vi "DO Monitoring Global Variables.vi"() -> ()   [LabVIEW 2014]
panel:
  in  "OutPuts":T1(tab)
  out "View Out":T2
  out "View Out 2":T2
  out "View Out 3":T2
  out "View Out 4":T2
  out "View Out 5":T2
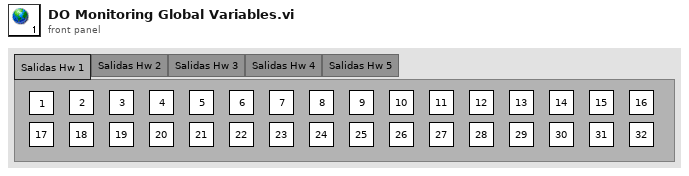
[diagram p1: front panel]
types:
  T1 = enum32{"Salidas Hw 1", "Salidas Hw 2", "Salidas Hw 3", "Salidas Hw 4", "Salidas Hw 5"}
  T2 = cluster{"Boolean 36":bool, "Boolean 3":bool, "Boolean 35":bool, "Boolean 34":bool, "Boolean 33":bool, "Boolean 32":bool, "Boolean 16":bool, "Boolean 17":bool, "Boolean 26":bool, "Boolean 25":bool, "Boolean 24":bool, "Boolean 23":bool, "Boolean 37":bool, "Boolean 1":bool, "Boolean 15":bool, "Boolean 4":bool, "Boolean 5":bool, "Boolean 6":bool, "Boolean 7":bool, "Boolean 8":bool, "Boolean 9":bool, "Boolean 10":bool, "Boolean 11":bool, "Boolean 12":bool, "Boolean 38":bool, "Boolean 21":bool, "Boolean 22":bool, "Boolean 20":bool, "Boolean 19":bool, "Boolean 18":bool, "Boolean 40":bool, "Boolean 39":bool}
diagram:
